vi "Test Worker Job Count Incremented.vi"(8 "error in (no error)":errorcluster, 11 "Cashier Test in":refnum<class "Cashier Test.lvclass">) -> (0 "error out":errorcluster, 3 "Cashier Test out":refnum<class "Cashier Test.lvclass">)   [LabVIEW 2020, in "Cashier Test.lvclass"]
uses:
  Cashier Test.lvclass
  C:/Users/anton/Documents/GitHub/Triarc-Examples/Coffee Shop/Worker Test/Worker Test.lvclass
  C:/Program Files (x86)/National Instruments/LabVIEW 2020/vi.lib/Asteme/LUnit/Test Case.lvclass
  Support/Beverages/TypeDefs/Drink Type.ctl
  Support/Beverages/TypeDefs/Options.ctl
  Customer/Customer.lvclass
  Stub Job Processor/Stub Job Processor.lvclass
  C:/Users/anton/Documents/GitHub/Triarc-Examples/Coffee Shop/Process Job/Job Handler.lvclass
  <vilib>/Asteme/Triarc Framework/Process/Process.lvclass/Process.ctl
  <vilib>/Asteme/LUnit/Test Case.lvclass/Test Case.ctl
  <vilib>/Asteme/LUnit/LUnit Assertion Result.lvclass/LUnit Assertion Result.ctl
  <vilib>/Asteme/Triarc Framework Test Suite/Support/Execution timer.vi
  <vilib>/Asteme/Triarc Framework/Process/Private/SubVIs/Wait for finish.vi
  <vilib>/Asteme/Triarc Framework/Process/Protected/Messaging/Enqueue Message.vi
  <vilib>/Asteme/Triarc Framework/Process/Private/SubVIs/Set Lifecycle State.vi
  <vilib>/Asteme/Triarc Framework/Process/Public/Lifecycle/Get Lifecycle State.vi
  <vilib>/Asteme/LUnit/Palette/Pass.vi
  <vilib>/Asteme/LUnit/Palette/Fail.vi
  <vilib>/Asteme/LUnit/Variant to string.vi
  <vilib>/Asteme/LUnit/Set Assertion Type.vi
  <vilib>/Utility/error.llb/Clear Errors.vi
  <vilib>/Asteme/LUnit/Add test result.vi
  <vilib>/Asteme/LUnit/LUnit Write Passed.vi
  <vilib>/Asteme/LUnit/LUnit Get Test Case.vi
  <vilib>/Asteme/LUnit/Assertion Result/LUnit Get Test Name.vi
  <vilib>/Asteme/LUnit/LUnit Write Message.vi
  <vilib>/Asteme/LUnit/LUnit Write Description.vi
  <vilib>/Asteme/LUnit/LUnit Write Assertion Type.vi
  <vilib>/Asteme/LUnit/Read Test Case Name.vi
  Worker/Worker.lvclass
  C:/Program Files (x86)/National Instruments/LabVIEW 2020/vi.lib/Asteme/Triarc Framework/Process/Process.lvclass
  <vilib>/Asteme/Triarc Framework Test Suite/Support/Event Helpers/Dequeue Event Message.vi
  <vilib>/Utility/error.llb/Error Cluster From Error Code.vi
  <vilib>/Utility/Data Type/Get Type Information.vi
  <vilib>/Utility/LVClass/Get LV Class Name.vi
  <vilib>/Asteme/LUnit/LUnit Assertion Result.lvclass
  <vilib>/Asteme/Triarc Framework/Process/Process.lvclass
  Worker Test/Worker Test.lvclass
  <vilib>/Asteme/LUnit/Test Case.lvclass
  <vilib>/Asteme/Triarc Framework Test Suite/Support/Event Helpers/Event Helpers.lvlib
  Support/Order/Order.lvclass
  Support/Beverages/Beverage/Beverage.lvclass
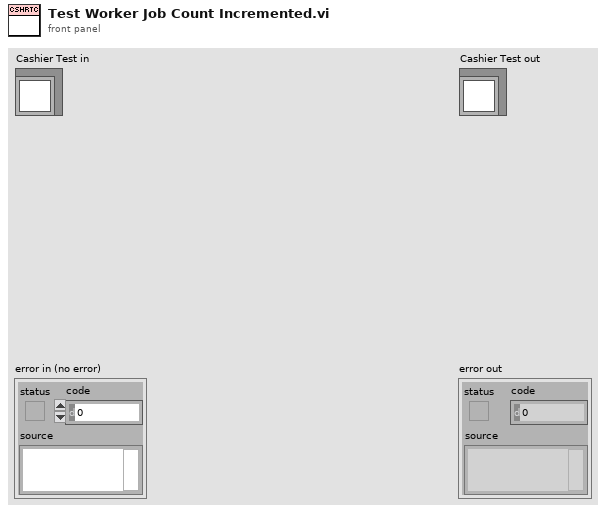
[diagram p1: front panel]
types:
  T1 = typedef "Beverage.lvclass/Drink Type.ctl" = enum16{"Dark Roast", "Decaf", "Espresso", "House Blend"}
  T2 = typedef "Beverage.lvclass/Options.ctl" = enum16{"<None>", "Milk", "Mocha", "Soy", "Whip"}
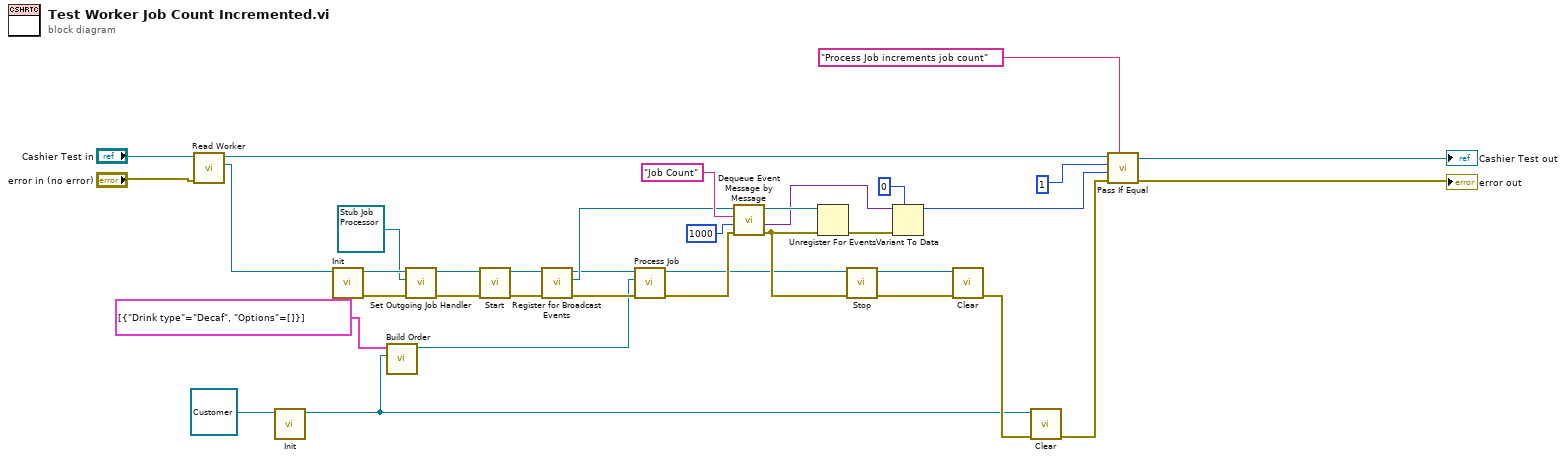
[diagram p0: block diagram]
diagram:
  n1 = call "Read Worker.vi"("error in (no error)"="error in (no error)", "Worker Test in"="Cashier Test in") -> ("Worker"=w12:refnum<class "Worker.lvclass">, "Worker Test out"=w11:refnum<class "Cashier Test.lvclass">)  [unwired: 7 in, 1 out]
  n2 = call-dynamic "Init.vi"("View In"=refnum<class "Customer.lvclass"> refnum ("Customer.lvclass")) -> ("View Out"=w6:refnum<class "Customer.lvclass">)  [unwired: 9 in, 1 out]
  n3 = call-dynamic "Init.vi"("View In"=w12) -> ("error out"=w13:errorcluster, "View Out"=w3:refnum<class "Worker.lvclass">)  [unwired: 9 in]
  n4 = call "Build Order.vi"("Customer"=w6, "Order"=cluster{"Drink type":T1, "Options":T2[]}[] [{"Drink type"=enum."Decaf", "Options"=[]}]) -> ("Order Out"=w5:refnum<class "Order.lvclass">)  [unwired: 7 in, 2 out]
  n5 = call "Set Outgoing Job Handler.vi"("error in (no error)"=w13, "Work Dispatcher"=refnum<class "Stub Job Processor.lvclass"> refnum ("Stub Job Processor.lvclass"), "Worker In"=w3) -> ("error out"=w4:errorcluster, "Worker Out"=w2:refnum<class "Worker.lvclass">)  [unwired: 7 in]
  n6 = call <vilib>:"Start.vi"("error in (no error)"=w4, "Process In"=w2) -> ("error out"=w16:errorcluster, "Process Out"=w19:refnum<class "Worker.lvclass">)  [unwired: 8 in]
  n7 = call <vilib>:"Register for Broadcast Events.vi"("error in (no error)"=w16, "Process In"=w19) -> ("error out"=w18:errorcluster, "Event Registration Refnum Out"=w23:refnum<event-registration>, "Process Out"=w20:refnum<class "Worker.lvclass">)  [unwired: 7 in]
  n8 = call-dynamic "Process Job.vi"("error in (no error)"=w18, "Task"=w5, "Worker In"=w20) -> ("error out"=w22:errorcluster, "Worker Out"=w21:refnum<class "Worker.lvclass">)  [unwired: 7 in]
  n9 = call <vilib>:"Dequeue Event Message by Message.vi"("error in (no error)"=w22, "Timeout (-1)"=1000, "Message"="Job Count", "Event Registration Refnum"=w23) -> ("error out"=w29:errorcluster, "Message Data"=w26:variant, "Event Registration Refnum Out"=w32:refnum<event-registration>)  [unwired: 3 in, 2 out]
  n10 = Unregister For Events(event registration refnum=w32, error in=w29) -> (error out=w31:errorcluster)
  n11 = call <vilib>:"Stop.vi"("error in (no error)"=w29, "Process In"=w21) -> ("error out"=w15:errorcluster, "Process Out"=w14:refnum<class "Worker.lvclass">)  [unwired: 7 in, 1 out]
  n12 = Variant To Data(error in=w31, type=u32 0 ("code"), Variant=w26) -> (data=w28:u32)  [unwired: 1 out]
  n13 = call-dynamic "Clear.vi"("error in (no error)"=w15, "View In"=w14) -> ("error out"=w8:errorcluster)  [unwired: 9 in]
  n14 = call-dynamic "Clear.vi"("error in (no error)"=w8, "View In"=w6) -> ("error out"=w7:errorcluster)  [unwired: 9 in]
  n15 = call <vilib>:"Pass If Equal.vi"("Description"="Process Job increments job count", "error in (no error)"=w7, "Actual"=w28, "Expected"=u32 1 ("code"), "Test Case In"=w11) -> ("error out"=→"error out":errorcluster, "Test Case Out"=→"Cashier Test out":refnum<class "Cashier Test.lvclass">)  [unwired: 5 in]
